vi "Update Progress Bar.vi"(6 "Current Iteration":i32, 8 "error in":errorcluster, 10 "Expected iterations":i32=4, 11 "Queue in":refnum<queue>) -> (0 "error out":errorcluster, 1 "Message":string, 2 "Progress":i32, 3 "Queue out":refnum<queue>, 4 "Stop?":bool)   [LabVIEW 2016, in "Server Controller.lvlib" / "Server Controller.lvclass"]
uses:
  Server Controller.lvclass
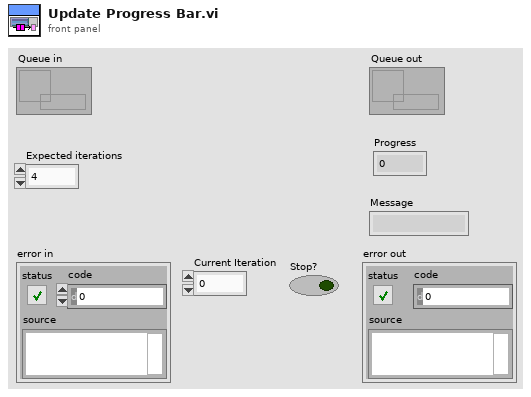
[diagram p1: front panel]
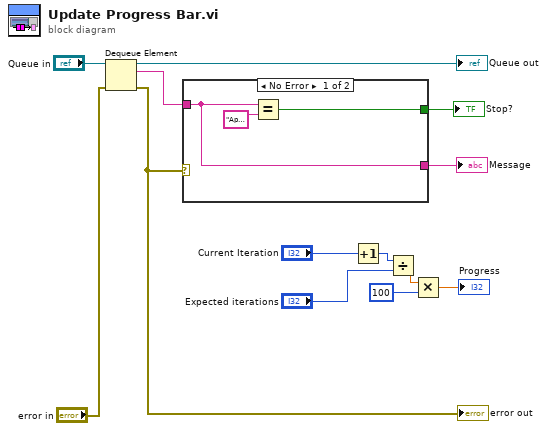
[diagram p0: block diagram]
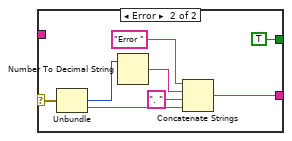
[diagram p2: hidden frame]
diagram:
  n1 = Dequeue Element(queue="Queue in", error in (no error)="error in") -> (queue out=→"Queue out":refnum<queue>, element=w9:string, error out=w10:errorcluster)  [unwired: 1 in, 1 out]
  "error out" <- w10
  n2 = case shown="No Error" w10 {
    selector: w10 -> [_ w24]
    tunnel: w9 -> [w14 _]
    tunnel: [w14 w18] -> w7
    tunnel: [w15 TRUE] -> w8
    frame No Error {
      n3 = Equal?(x=w14, y="Application is broken and cannot be run." ("notification")) -> (x = y?=w15:bool)
    }
    frame Error {
      n4 = Unbundle(w24) -> ("code"=w22:i32, "source"=w23:string)  [unwired: 1 out]
      n5 = Number To Decimal String(number=w22) -> (decimal integer string=w21:string)  [unwired: 1 in]
      n6 = Concatenate Strings("Error " ("string"), w21, ". " ("string"), w23) -> (w18:string)
    }
  }
  "Stop?" <- w8
  "Message" <- w7
  n7 = Increment(x="Current Iteration") -> (x+1=w4:i32)
  n8 = Divide(x=w4, y="Expected iterations") -> (x/y=w6:dbl)
  n9 = Multiply(x=w6, y=100) -> (x*y=→"Progress":dbl)
